vi "624WPI_DashboardAdjust Dashboard Window.vi"(8 "height":i32, 9 "width":i32, 10 "reference in":refnum<vi>, 11 "Notifier in":refnum<notifier>) -> ()   [LabVIEW 2013]
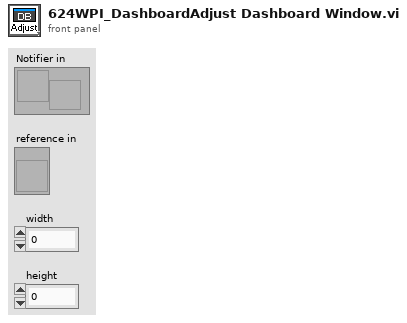
[diagram p1: front panel]
types:
  T1 = typedef "LVRectTypeDef.ctl" = cluster{"Left":i16, "Top":i16, "Right":i16, "Bottom":i16}
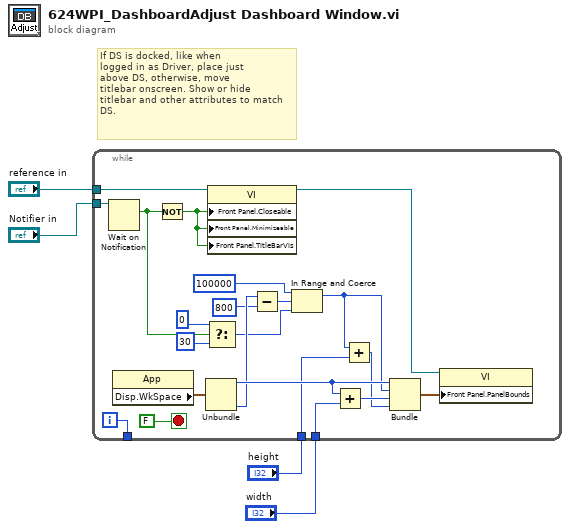
[diagram p0: block diagram]
diagram:
  # "If DS is docked, like when\nlogged in as Driver, place just\nabove DS, otherwise, move\ntitlebar onscreen. Show or hide\ntitlebar and other attributes to match\nDS."
  n1 = while {
    tunnel: "Notifier in" -> [w25]
    tunnel: [w24] -> _
    tunnel: "height" -> [w9]
    tunnel: "width" -> [w8]
    tunnel: "reference in" -> [w6]
    i -> [w24]
    stop <- FALSE stop-if-true
    n2 = Wait on Notification(notifier=w25) -> (notification=w13:bool)  [unwired: 3 in, 3 out]
    n3 = property class="App"() -> ("Disp.WkSpace"=w22:T1)  [unwired: 2 in, 2 out]
    n4 = Not(x=w13) -> (.not. x?=w5:bool)
    n5 = Unbundle(w22) -> ("Left"=w20:i16, "Bottom"=w18:i16)  [unwired: 2 out]
    n6 = Select(t=0, s=w13, f=30) -> (s? t:f=w12:i32)
    n7 = property class="VI"(reference=w6, "Front Panel.Closeable"=w5, "Front Panel.Minimizeable"=w5, "Front Panel.TitleBarVis"=w5) -> (reference out=w7:refnum<vi>)  [unwired: 1 in, 1 out]
    n8 = Subtract(x=w18, y=800) -> (x-y=w16:i32)
    n9 = In Range and Coerce(upper limit=100000, x=w16, lower limit=w12) -> (coerced(x)=w10:i32)  [unwired: 1 out]
    n10 = Add(x=w20, y=w8) -> (x+y=w21:i32)
    n11 = Add(x=w10, y=w9) -> (x+y=w19:i32)
    n12 = Bundle("Left"=w20, w10, w21, w19) -> (w23:cluster{"Left":i16, i32, i32, i32})  [unwired: 1 out]
    n13 = property class="VI"(reference=w7, "Front Panel.PanelBounds"=w23) -> ()  [unwired: 1 in, 2 out]
  }
